vi "Interpolate Y (multiple).vi"(8 "error in (no error)":errorcluster, 10 "x (0)":dbl, 11 "XY-data":cluster{"X-array":dbl[], "Y-array":dbl[]}[](array[cluster])) -> (0 "error out":errorcluster, 2 "y":dbl[](array[numeric]), 3 "XY-data out":cluster{"X-array":dbl[], "Y-array":dbl[]}[](array[cluster]) {"Y-array" format="%.2p"; "X-array" format="%.2p"})   [LabVIEW 2019, in "xy_utilities.lvlib"]
doc: "Given a fractional <b>x</b> value, interpolate a factional <b>y</b> value.\n\nWire data to the data input to determine the polymorphic instance to use or manually select the instance."
uses:
  xy_utilities.lvlib
  Sort.vi
  Sort (single).vi
  <userlib>/_OpenG.lib/array/array.llb/Sort Array__ogtk.vi
  <userlib>/_OpenG.lib/array/array.llb/Sort 1D Array (DBL)__ogtk.vi
  <userlib>/_OpenG.lib/array/array.llb/Reorder Array2__ogtk.vi
  <userlib>/_OpenG.lib/array/array.llb/Reorder 1D Array2 (DBL)__ogtk.vi
  <userlib>/_MGI/1D Array/MGI Threshold 1D Array Extended.vi
  <userlib>/_MGI/1D Array/MGI Interpolate 1D Array Extended.vi
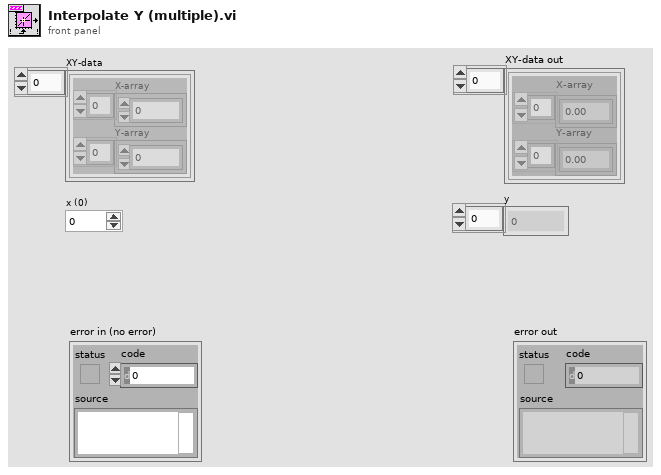
[diagram p1: front panel]
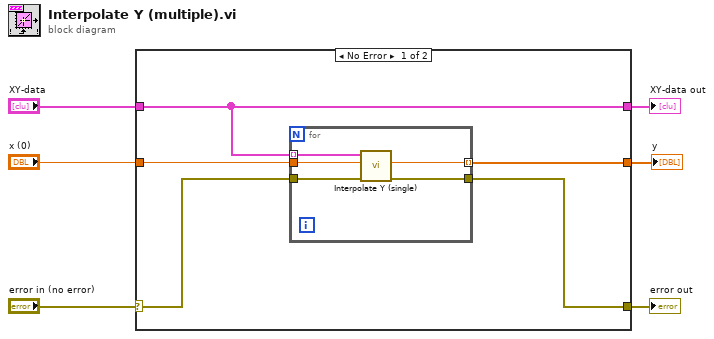
[diagram p0: block diagram]
diagram:
  n1 = case shown="No Error" "error in (no error)" {
    selector: "error in (no error)" -> [w11 w18]
    tunnel: [w8 w18] -> w5
    tunnel: "XY-data" -> [w7 w17]
    tunnel: [w7 w17] -> w3
    tunnel: "x (0)" -> [w10 _]
    tunnel: [w9 _] -> w1
    frame No Error {
      n2 = for {
        tunnel: w11 -> [w16]
        tunnel: w10 -> [w15]
        tunnel: w7 -> [w14] mode=indexing
        tunnel: [w13] -> w9 mode=indexing
        tunnel: [w12] -> w8
        n3 = call "Interpolate Y (single).vi"("error in (no error)"=w16, "x (0)"=w15, "XY-data"=w14) -> ("error out"=w12:errorcluster, "y"=w13:dbl)  [unwired: 6 in, 1 out]
      }
    }
    frame Error {
    }
  }
  "error out" <- w5
  "XY-data out" <- w3
  "y" <- w1
